vi "20151027 accel+gyro average for offset .vi"() -> ()   [LabVIEW 2013]
uses:
  <vilib>/MakerHub/LINX/Public/Sensors/Accelerometer/MPU60X0/DeviceAddresses.ctl
  <vilib>/MakerHub/LINX/Public/Sensors/Accelerometer/MPU60X0/AccelFullScaleRanges.ctl
  <vilib>/MakerHub/LINX/Public/Sensors/Accelerometer/MPU60X0/GyroFullScaleRanges.ctl
  <vilib>/MakerHub/LINX/Public/Sensors/Accelerometer/MPU60X0/MPU60X0.lvlib
  <vilib>/MakerHub/LINX/LMH-LINX.lvlib
panel:
  out "Gz":dbl
  out "Gy":dbl
  out "Gx":dbl
  out "Accz":dbl
  out "Accy":dbl
  out "Accx":dbl
  out "Elapsed time":u32
  out "Temperature (°C)":dbl
  out "Gyro":T1(graph)
  out "Accel":T1(graph)
  in  "Serial Port":refnum<visa-resource-name>="COM10"
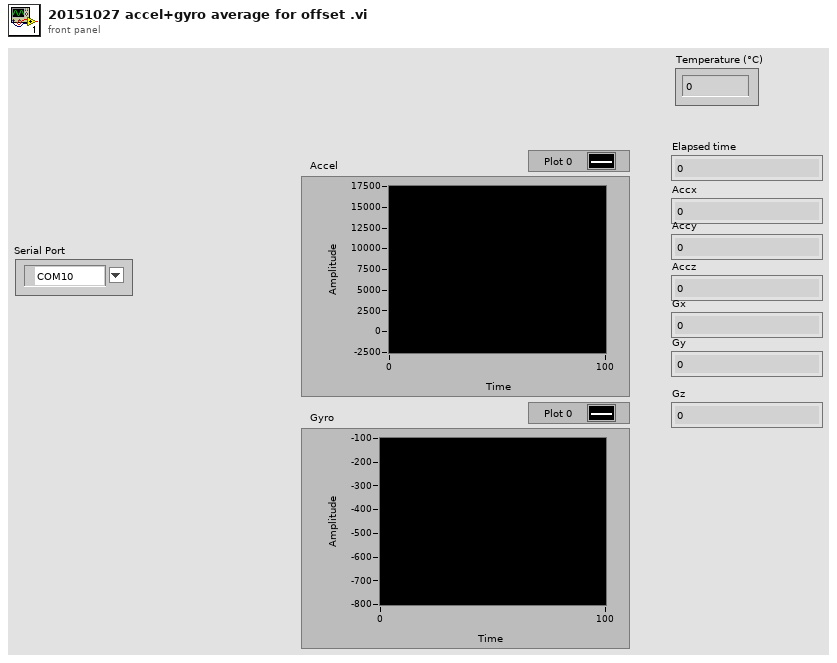
[diagram p1: front panel]
types:
  T1 = cluster{"X Axis":i16, "Y Axis":i16, "Z Axis":i16}
  T2 = typedef "LMH-LINX.lvlib/MPU60X0.lvlib/GyroFullScaleRanges.ctl" = enum8{"±250 °/s", "±500 °/s", "±1000 °/s", "±2000 °/s"}
  T3 = typedef "LMH-LINX.lvlib/MPU60X0.lvlib/AccelFullScaleRanges.ctl" = enum16{"±2g", "±4g", "±8g", "±16g"}
  T4 = typedef "LMH-LINX.lvlib/MPU60X0.lvlib/DeviceAddresses.ctl" = enum16{"0x68", "0x69"}
  T5 = typedef "LMH-LINX.lvlib/LINX Ref.ctl" = cluster{"Platform":T6, "Interface":T7, "LINX Device Config":T8}
  T6 = typedef "LMH-LINX.lvlib/Platform.ctl" = enum16{"LINX", "myRIO"}
  T7 = typedef "LMH-LINX.lvlib/Interface.ctl" = enum16{"Serial", "TCP"}
  T8 = typedef "LMH-LINX.lvlib/Device.lvlib/LINX Device Config.ctl" = cluster{"Interface":T7, "COM Port":refnum<visa-resource-name>, "TCP Configuration":T9, "Device Family":u8, "Device ID":u8, "Device Name":string, "TCP Ref":refnum<k5>, "Channels":T10}
  T9 = typedef "LMH-LINX.lvlib/Device.lvlib/TCP Config.ctl" = cluster{"IP Address":string, "Port":u16}
  T10 = typedef "LMH-LINX.lvlib/Channels.ctl" = cluster{"DI":u8[], "DO":u8[], "AI":u8[], "AO":u8[], "PWM":u8[], "QE":u8[], "UART":u8[], "I2C 2":u8[], "SPI":u8[], "CAN":u8[], "Servo":u8[], "AI Ref (V)":dbl, "AO Ref (V)":dbl, "AO Resolution (Bits)":u8}
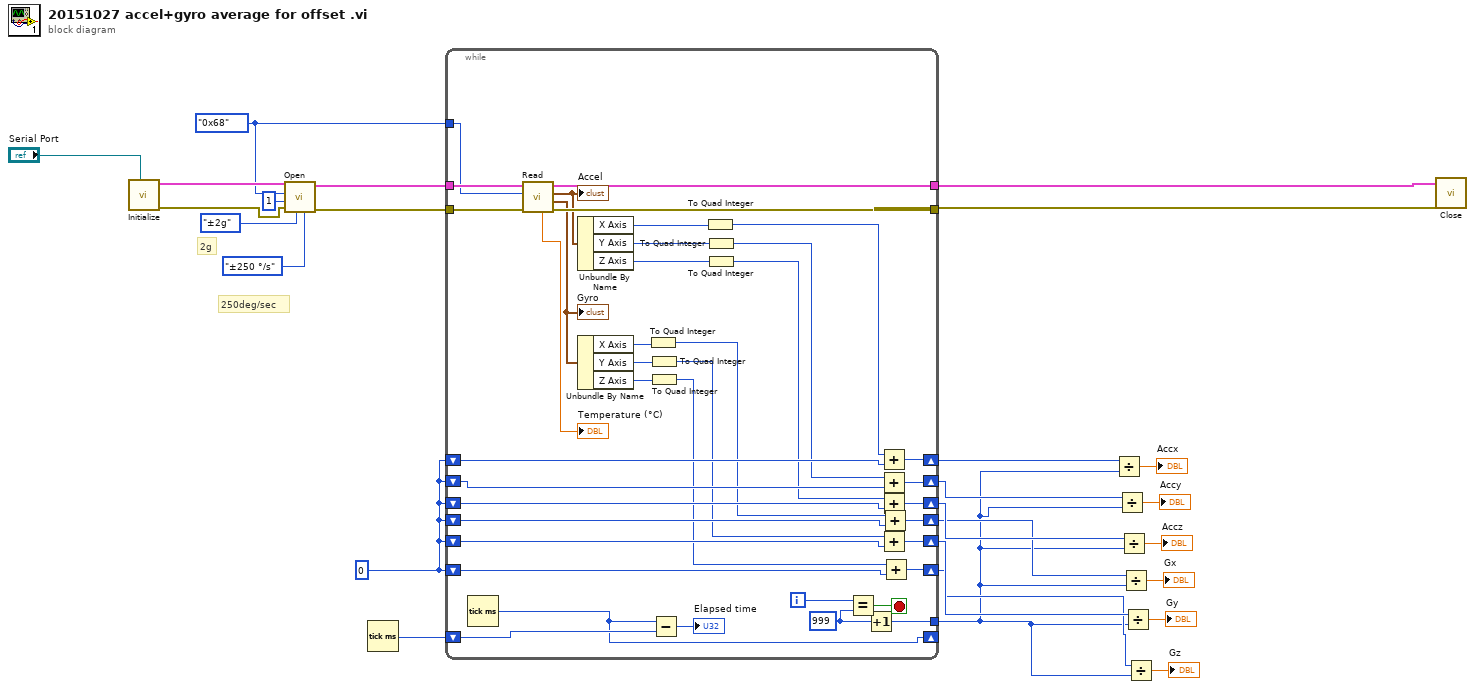
[diagram p0: block diagram]
diagram:
  w14 = i64 0
  w21 = DeviceAddresses."0x68" ("Device Address")
  # "250deg/sec"
  # "2g"
  n1 = call <vilib>:"Initialize.vi"("Serial Port"="Serial Port") -> ("Error Out"=w23:errorcluster, "LINX Ref"=w24:T5)  [unwired: 8 in, 1 out]
  n2 = call <vilib>:"Open.vi"("Gyro Full Scale Range"=GyroFullScaleRanges."±250 °/s", "Accel Full Scale Range"=AccelFullScaleRanges."±2g", "Error In"=w23, "Clock Source"=u8 1, "Device Address"=w21, "LINX Resource"=w24) -> ("Error Out"=w25:errorcluster, "LINX Resource"=w26:T5)  [unwired: 4 in]
  n3 = Tick Count (ms)() -> (millisecond timer value=w16:u32)
  n4 = while {
    tunnel: w26 -> [w65]
    tunnel: w25 -> [w64]
    tunnel: [w63] -> w20
    tunnel: [w62] -> w19
    tunnel: w21 -> [w61]
    shift-right: [w57] -> w2
    shift-left: w14 -> [w56]
    shift-right: [w54] -> _
    shift-left: w16 -> [w55]
    shift-right: [w53] -> w3
    shift-left: w14 -> [w44]
    shift-right: [w52] -> w4
    shift-left: w14 -> [w45]
    shift-right: [w51] -> w5
    shift-left: w14 -> [w46]
    shift-right: [w50] -> w6
    shift-left: w14 -> [w47]
    shift-right: [w49] -> w13
    shift-left: w14 -> [w48]
    tunnel: [w27] -> w1
    i -> [w29]
    stop <- w30 stop-if-true
    w28 = 999 ("y")
    n5 = Tick Count (ms)() -> (millisecond timer value=w54:u32)
    n6 = call <vilib>:"Read.vi"("Error In"=w64, "Device Address"=w61, "LINX Resource"=w65) -> ("Error Out"=w62:errorcluster, "Gyro  Data"=w59:T1, "Acceleration Data"=w60:T1, "LINX Resource"=w63:T5, "Temperature (°C)"=→"Temperature (°C)":dbl)  [unwired: 4 in]
    "Accel" <- w60
    "Gyro" <- w59
    n7 = Unbundle By Name(w60) -> ("X Axis"=w43:i16, "Y Axis"=w41:i16, "Z Axis"=w39:i16)
    n8 = Unbundle By Name(w59) -> ("X Axis"=w36:i16, "Y Axis"=w35:i16, "Z Axis"=w37:i16)
    n9 = To Quad Integer(1:w36) -> (0:w34:i64)
    n10 = To Quad Integer(1:w35) -> (0:w33:i64)
    n11 = To Quad Integer(1:w37) -> (0:w32:i64)
    n12 = Subtract(x=w54, y=w55) -> (x-y=→"Elapsed time":u32)
    n13 = To Quad Integer(1:w43) -> (0:w42:i64)
    n14 = To Quad Integer(1:w41) -> (0:w40:i64)
    n15 = To Quad Integer(1:w39) -> (0:w38:i64)
    n16 = Equal?(x=w29, y=w28) -> (x = y?=w30:bool)
    n17 = Increment(x=w28) -> (x+1=w27:i32)
    n18 = Add(x=w42, y=w48) -> (x+y=w49:i64)
    n19 = Add(x=w40, y=w47) -> (x+y=w50:i64)
    n20 = Add(x=w38, y=w46) -> (x+y=w51:i64)
    n21 = Add(x=w33, y=w44) -> (x+y=w53:i64)
    n22 = Add(x=w34, y=w45) -> (x+y=w52:i64)
    n23 = Add(x=w32, y=w56) -> (x+y=w57:i64)
  }
  n24 = Divide(x=w13, y=w1) -> (x/y=→"Accx":dbl)
  n25 = Divide(x=w6, y=w1) -> (x/y=→"Accy":dbl)
  n26 = Divide(x=w5, y=w1) -> (x/y=→"Accz":dbl)
  n27 = Divide(x=w4, y=w1) -> (x/y=→"Gx":dbl)
  n28 = Divide(x=w3, y=w1) -> (x/y=→"Gy":dbl)
  n29 = Divide(x=w2, y=w1) -> (x/y=→"Gz":dbl)
  n30 = call <vilib>:"Close.vi"("Error In"=w19, "LINX Resource"=w20) -> ()  [unwired: 8 in, 2 out]
